vi "WS PuTTY Tool.vi"() -> ()   [LabVIEW 2015]
uses:
  NationalInstruments.VeriStand.SystemStorage
  NationalInstruments.VeriStand.SystemDefinitionAPI
panel:
  in  "NIVS.System Definition Root":refnum<k24>
  in  "NIVS.Project File Path":path
  in  "NIVS.Workspace Event":refnum<event-registration>
  in  "NIVS.Gateway IP Address":string
  in  "NIVS.INI File Path":path
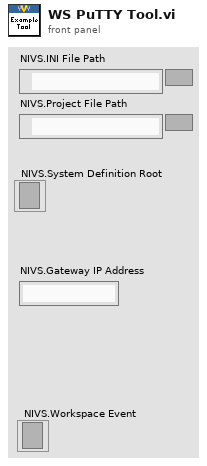
[diagram p1: front panel]
types:
  T1 = enum8{"open", "edit", "explore", "find", "print"}
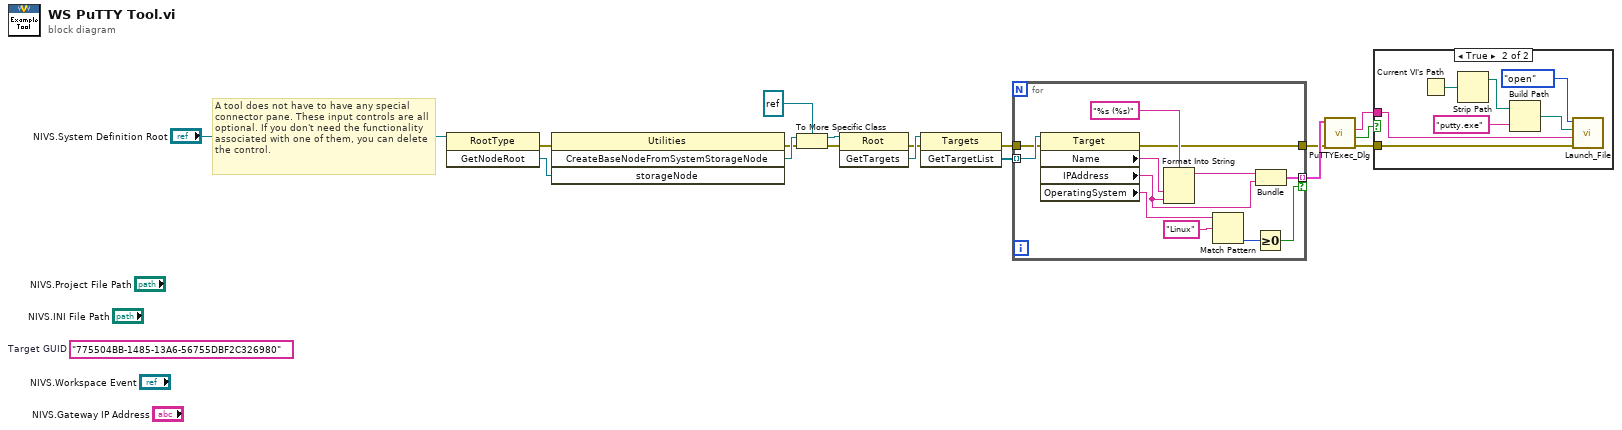
[diagram p0: block diagram]
diagram:
  (unwired) "775504BB-1485-13A6-56755DBF2C326980"  # Target GUID
  # "A tool does not have to have any special connector pane. These input controls are all optional. If you don't need the functionality associated with one of them, you can delete the control."
  n1 = invoke class="RootType" method="GetNodeRoot"(reference="NIVS.System Definition Root") -> (error out=w1:errorcluster, "GetNodeRoot"=w16:refnum<k24>)  [unwired: 2 in, 1 out]
  n2 = invoke class="Utilities" method="CreateBaseNodeFromSystemStorageNode"(error in=w1, "storageNode"=w16) -> (error out=w2:errorcluster, "CreateBaseNodeFromSystemStorageNode"=w15:refnum<k24>)  [unwired: 2 in, 2 out]
  n3 = To More Specific Class(target class=refnum<k24> refnum, reference=w15, error in=w2) -> (specific class reference=w13:refnum<k24>, error out=w3:errorcluster)
  n4 = invoke class="Root" method="GetTargets"(reference=w13, error in=w3) -> (error out=w4:errorcluster, "GetTargets"=w12:refnum<k24>)  [unwired: 1 in, 1 out]
  n5 = invoke class="Targets" method="GetTargetList"(reference=w12, error in=w4) -> (error out=w5:errorcluster, "GetTargetList"=w11:refnum<k24>[])  [unwired: 1 in, 1 out]
  n6 = for {
    tunnel: w11 -> [w29] mode=indexing
    tunnel: [w22] -> w10 mode=indexing if=w20
    tunnel: [w19] -> w6
    tunnel: w5 -> [w18]
    n7 = property class="Target"(reference=w29, error in=w18) -> (error out=w19:errorcluster, "Name"=w24:string, "IPAddress"=w23:string, "OperatingSystem"=w27:string)  [unwired: 1 out]
    n8 = Format Into String(format string="%s (%s)", w24, w23) -> (resulting string=w25:string)  [unwired: 2 in, 1 out]
    n9 = Match Pattern(string=w27, regular expression="Linux") -> (offset past match=w21:i32)  [unwired: 1 in, 3 out]
    n10 = Greater Or Equal To 0?(x=w21) -> (x >= 0?=w20:bool)
    n11 = Bundle(w25, "IPAddress"=w23) -> (w22:cluster{string, "IPAddress":string})  [unwired: 1 in]
  }
  n12 = call "PuTTYExec_Dlg.vi"("error in (no error)"=w6, "Targets Info"=w10) -> ("error out"=w7:errorcluster, "Open PuTTY Out"=w9:bool, "Parameters"=w8:string)  [unwired: 7 in]
  n13 = case shown="True" w9 {
    tunnel: w8 -> [_ w31]
    tunnel: w7 -> [_ w30]
    frame False {
    }
    frame True {
      n14 = Current VI's Path() -> (path=w34:path)
      n15 = Strip Path(path=w34) -> (stripped path=w35:path)  [unwired: 1 out]
      n16 = Build Path(base path=w35, name or relative path="putty.exe") -> (appended path=w33:path)
      n17 = call "Launch_File.vi"("error in"=w30, "Parameters"=w31, "path"=w33, "Operation"=T1."open") -> ()  [unwired: 5 in, 1 out]
    }
  }
